vi "HEWH Gas Thermal Rate Tester.vi"() -> ()   [LabVIEW 2019]
uses:
  Type Definitions/HEWH Output Information.ctl
  Type Definitions/HEWH Draw Pattern Setup.ctl
  Type Definitions/PRAT Test.ctl
  Utility/Save File/File Setup (Public)/Type Definition/Save File HEWH Heating Control Mode.ctl
  Support VIs/Draw Water Specific/Type Definitions/Terminate Draw Conditions.ctl
  Type Definitions/HEWH Start Conditions.ctl
  Support VIs/Draw Water Specific/Type Definitions/Check Special Condtions.ctl
  Support VIs/Draw Water Specific/Type Definitions/HEWH Special Condition Check.ctl
  Type Definitions/HEWH Draw Flag ENUM.ctl
  Type Definitions/HEWH Specific DAQ.ctl
  Type Definitions/HEWH Power Data.ctl
  Type Definitions/HEWH Power Elements.ctl
  Utility/Type Definitions/UTILITY Power Analyzer.ctl
  Type Definitions/HEWH Calc and Calibration.ctl
  Utility/Save File/File Setup (Public)/Type Definition/Save File DOE LabView Program.ctl
  Custom Instrument Control/MW100/Type Definitions/Station ID Selector.ctl
  Range/Type Definitions/RANGE ANSI Rate.ctl
  Drivers/Alicat Gas Meter Driver/Sub-VIs/Data Cluster.ctl
  <vilib>/Utility/file.llb/Read Delimited Spreadsheet (string).vi
  Utility/Save File/File Setup.lvlib
panel:
  out "Target Flow Rate (GPM)":dbl
  out "States":T1(array[ring])
  in  "FileInit Cluster Input in":T2={"Scan Rate Adjust"=0.0, "Draw Count"=0, "Test Patten Setup"={"Total Gallons Schedule"=[], "PRAT/RLT Sequence"=[], "Current Sequence Index"=0}, "HEWH Specific DAQ"={"HEWH Data"={"HEWH Standard"={"Voltage (Volts)"=0.0, "Current (Amps)"=0.0, "Power (Watts)"=0.0, "WattHours (Wh)"=0.0, "TC Tree (AVG)"=0.0, "Flow Rate (GPM)"=0.0, "Gallons (Gal)"=0.0, "RTD Out (Deg F)"=0.0, "RTD In (Deg F)"=0.0, "RTD Amb (Deg F)"=0.0, "TC Down"=0.0, "UE Event Lead"=0, "LE Event Lead"=0, "TC Tree Array"=[]}, "PRAT"={"Power (Watts) A"=0.0, "Power (Watts) B"=0.0, "Power (Watts) C"=0.0, "Power (Watts) D"=0.0, "TC1"=0.0, "TC2"=0.0, "TC3"=0.0, "TC4"=0.0, "WattHours (Wh) A"=0.0, "WattHours (Wh) B"=0.0, "WattHours (Wh) C"=0.0, "WattHours (Wh) D"=0.0, "Ambient"=0.0, "Extra Temp"=0.0}, "Additional Power Data"={"Vthd"=0.0, "Frequency (Hz)"=0.0, "Apparent Power (VA)"=0.0, "Power Factor"=0.0, "Current Crest Factor"=0.0, "Voltage Crest Factor"=0.0, "Integration Time (sec)"=0.0}}, "Flow Valve % Open"=0.0, "Power State"={"UE"=FALSE, "LE"=FALSE, "COMP"=FALSE, "FANS"=FALSE}, "Power Analyzer"=enum."", "Flow Valve uA Output"=0, "Gallons Start (Gal)"=0.0}, "Test Output Data"={"PreDraw Data Table"=[], "Data Table"=[], "MW100 TC Headers"=[]}, "Calc and Calibration"={"Mean SD Var Max Min Array"=[], "Draw Statistics (DBL)"=[], "Calibration Coefficients DBL"=[], "Start Gallons"=0.0, "Starting Temp Decline"=0.0, "K-Factor (Temperature)"=0.0, "All Draw Stats"=[], "RTD Terminate Value"=0.0, "K-Factor (Flow)"=0.0, "Intellifaucet Type"="", "Gas Thermal Stabilization Array"=[], "Gas Thermal Stabil Complete"=FALSE, "Gas Thermal Time"=0.0, "Therm Reset Cmpt 1"=FALSE, "Therm Reset Cmpt 2"=FALSE, "Last Flow Rate (Therm)"=0.0, "State"=enum."State 1", "Gas Thermal Time 2"=0.0}, "Current Draw Time"=0.0, "LV Program"=enum."No Name Found", "Station ID"=enum."", "Current Cond"=enum."N/A", "Test Complete"=FALSE, "ANSI Rate"={"Array 1"=[], "Array 3"=[], "Array 2"=[], "Start ANSI"=FALSE, "ANSI Start Time"=0.0, "Restart ANSI"=FALSE, "15 Min ANSI Avg (BTU/hr)"=0.0, "20 Min ANSI Avg (BTU/hr)"=0.0, "25 Min ANSI Avg (BTU/hr)"=0.0, "Absolute Pressure"=0.0, "Gas Temperature"=0.0, "Volumetric Flow Rate"=0.0, "Mass Flow Rate"=0.0, "Array 4"=[], "Array 5"=[], "Gas Rate"=0.0, "15 Min Pres Avg (PSIA)"=0.0, "20 Min Pres Avg (PSIA)"=0.0, "25 Min Pres Avg (PSIA)"=0.0, "15 Min Temp Avg (°F) "=0.0, "20 Min Temp Avg (°F)"=0.0, "25 Min Temp Avg (°F)"=0.0, "15 Min Uncorrected Avg (CFH)"=0.0, "20 Min Uncorrected Avg (CFH)"=0.0, "25 Min Uncorrected Avg (CFH)"=0.0, "15 Min Corrected Avg (SCFH)"=0.0, "20 Min Corrected Avg (SCFH)"=0.0, "25 Min Corrected Avg (SCFH)"=0.0, "15 Min Complete"=FALSE, "20 Min Complete"=FALSE, "25 Min Complete"=FALSE, "Heating Value (BTU/ft³)"=0.0}, "Gas Measurment Data"={"Absolute Pressure"=0.0, "Gauge/Diff. Pressure"=0.0, "Barometric Pressure"=0.0, "Temperature"=0.0, "Volumetric Flow"=0.0, "Mass Flow"=0.0, "Setpoint"=0.0, "Valve Drive"=0.0, "Totalizer"=0.0, "[hr]"=0.0, "[min]"=0.0, "[sec]"=0.0, "Totalizer Average Flow"=0.0, "Totalizer Peak Flow"=0.0, "Gas selected"=""}} {"Test Patten Setup"."PRAT/RLT Sequence"."Time" format="%<%H:%M:%S>t"; "Test Patten Setup"."Total Gallons Schedule" format="%.2f"}
  in  "file path (dialog if empty)":path
  out "all rows":string[][](array[string])
  # "Totalizer Timer"
  # "Draw Pattern Setup (24 Hour)"
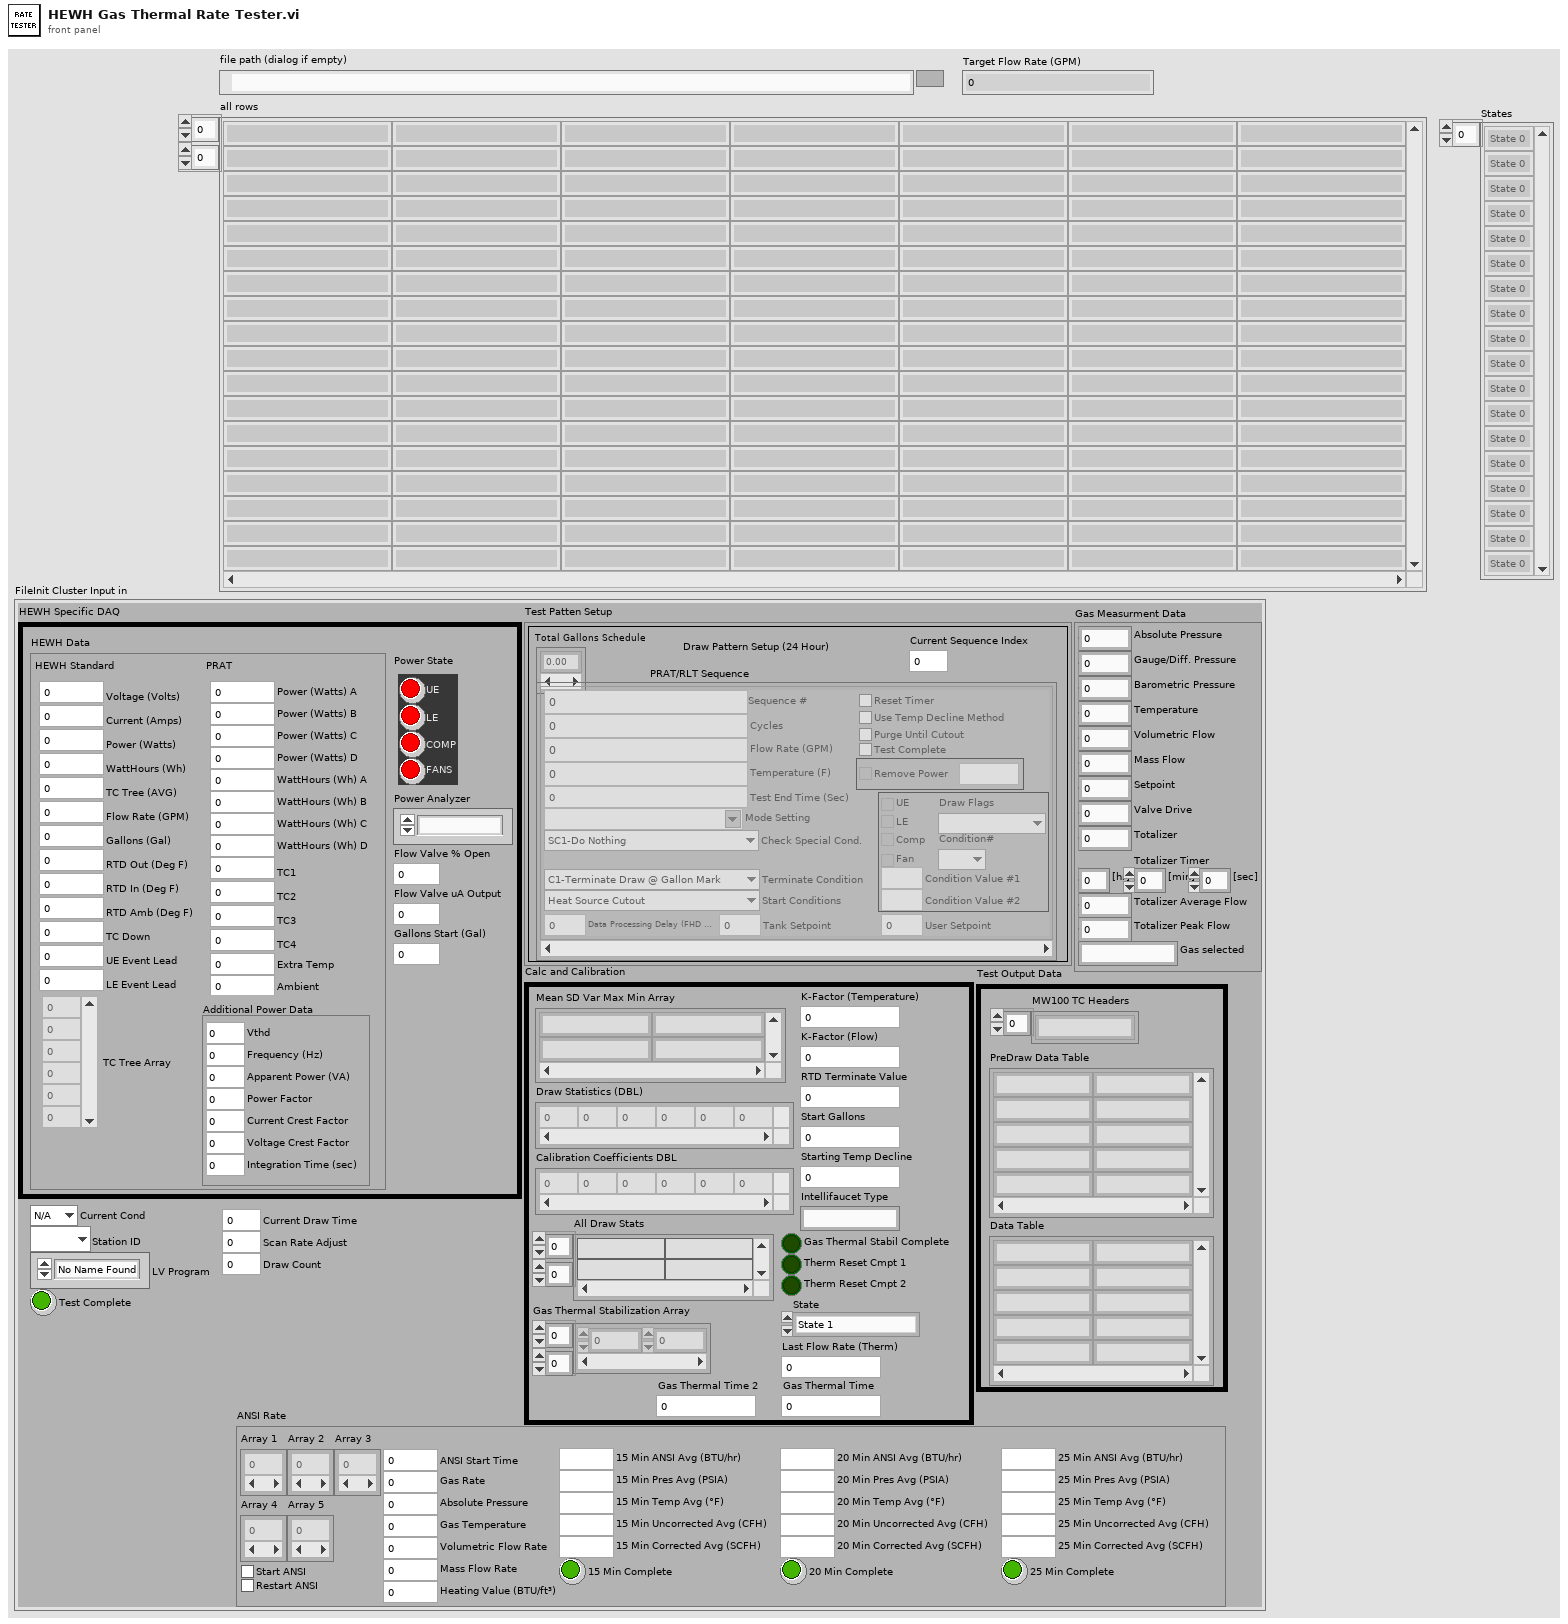
[diagram p1: front panel]
types:
  T1 = enum16{"State 0", "State 1", "State 2", "State 3", "State 4", "State 5"}[]
  T2 = typedef "HEWH Output Information.ctl" = cluster{"Scan Rate Adjust":dbl, "Draw Count":i32, "Test Patten Setup":T3, "HEWH Specific DAQ":T11, "Test Output Data":cluster{"PreDraw Data Table":string[][], "Data Table":string[][], "MW100 TC Headers":string[]}, "Calc and Calibration":T15, "Current Draw Time":dbl, "LV Program":T16, "Station ID":T17, "Current Cond":T9, "Test Complete":bool, "ANSI Rate":T18, "Gas Measurment Data":T19}
  T3 = typedef "HEWH Draw Pattern Setup.ctl" = cluster{"Total Gallons Schedule":dbl[], "PRAT/RLT Sequence":T4[], "Current Sequence Index":i32}
  T4 = typedef "PRAT Test.ctl" = cluster{"Sequence #":dbl, "Cycles":i32, "Mode Setting":T5, "Flow Rate (GPM)":dbl, "Temperature (F)":dbl, "Reset Timer":bool, "Use Temp Decline Method":bool, "Terminate Condition":T6, "Condition Value #1":dbl, "UE":bool, "LE":bool, "Comp":bool, "Fan":bool, "Test End Time (Sec)":dbl, "Purge Until Cutout":bool, "Start Conditions":T7, "Condition Value #2":dbl, "Remove Power":bool, "Time":dbl, "Check Special Cond.":T8, "Condition#":T9, "Draw Flags":T10, "Data Processing Delay (FHD 15sec, UEF 5 Sec)":dbl, "Test Complete":bool, "User Setpoint":dbl, "Tank Setpoint":dbl}
  T5 = typedef "File Setup.lvlib/Save File HEWH Heating Control Mode.ctl" = string
  T6 = typedef "Terminate Draw Conditions.ctl" = enum16{"C1-Terminate Draw @ Gallon Mark", "C2-Special Last Draw (HU Test)", "C3-RTD Out <=", "C4-Mean Tank Temp <=", "C5-Decrease RTD Out (Deg F)", "C6-Time (Seconds)", "C7-Until Any Heat Source", "C8-Specific Heat Source", "C9-Do Nothing", "C10-Inlet Outlet RTD Temp Delta"}
  T7 = typedef "HEWH Start Conditions.ctl" = enum16{"Heat Source Cutout", "At Time (Seconds)", "Every X (Seconds)", "T2 >= X° Below Setpoint", "Seconds From Complete", "Wait for LE & Comp Cutout", "Wait for Comp Cutout", "Wait for LE Cutout", "Wait for UE Cutout", "Start Immediately"}
  T8 = typedef "Check Special Condtions.ctl" = enum16{"SC1-Do Nothing", "SC2-Check Heat Source (On-C2/Off-C1)", "SC3-Check Skip Condition", "SC4-Check Heat Source ON/Fail", "SC5-Keep Draw Valves Open", "SC6-Skip Purge"}
  T9 = typedef "HEWH Special Condition Check.ctl" = enum16{"N/A", "C1", "C2", "Reset/Fail", "Skip Draw Sequence"}
  T10 = typedef "HEWH Draw Flag ENUM.ctl" = enum16{"N/A", "None(0)", "Sml(1)", "Med(2)", "SmlMed(3)", "Lrg(4)", "SmlLrg(5)", "MedLrg(6)", "SmlMedLrg(7)"}
  T11 = typedef "HEWH Specific DAQ.ctl" = cluster{"HEWH Data":T12, "Flow Valve % Open":dbl, "Power State":T13, "Power Analyzer":T14, "Flow Valve uA Output":i32, "Gallons Start (Gal)":dbl}
  T12 = typedef "HEWH Power Data.ctl" = cluster{"HEWH Standard":cluster{"Voltage (Volts)":dbl, "Current (Amps)":dbl, "Power (Watts)":dbl, "WattHours (Wh)":dbl, "TC Tree (AVG)":dbl, "Flow Rate (GPM)":dbl, "Gallons (Gal)":dbl, "RTD Out (Deg F)":dbl, "RTD In (Deg F)":dbl, "RTD Amb (Deg F)":dbl, "TC Down":dbl, "UE Event Lead":i32, "LE Event Lead":i32, "TC Tree Array":dbl[]}, "PRAT":cluster{"Power (Watts) A":dbl, "Power (Watts) B":dbl, "Power (Watts) C":dbl, "Power (Watts) D":dbl, "TC1":dbl, "TC2":dbl, "TC3":dbl, "TC4":dbl, "WattHours (Wh) A":dbl, "WattHours (Wh) B":dbl, "WattHours (Wh) C":dbl, "WattHours (Wh) D":dbl, "Ambient":dbl, "Extra Temp":dbl}, "Additional Power Data":cluster{"Vthd":dbl, "Frequency (Hz)":dbl, "Apparent Power (VA)":dbl, "Power Factor":dbl, "Current Crest Factor":dbl, "Voltage Crest Factor":dbl, "Integration Time (sec)":dbl}}
  T13 = typedef "HEWH Power Elements.ctl" = cluster{"UE":bool, "LE":bool, "COMP":bool, "FANS":bool}
  T14 = typedef "UTILITY Power Analyzer.ctl" = enum16{"", "APLUS", "WT210", "WT500", "WT300", "OSI", "Debug", "WT230", "WT300_1", "WT300_2"}
  T15 = typedef "HEWH Calc and Calibration.ctl" = cluster{"Mean SD Var Max Min Array":string[][], "Draw Statistics (DBL)":dbl[][], "Calibration Coefficients DBL":dbl[][], "Start Gallons":dbl, "Starting Temp Decline":dbl, "K-Factor (Temperature)":dbl, "All Draw Stats":string[][], "RTD Terminate Value":dbl, "K-Factor (Flow)":dbl, "Intellifaucet Type":string, "Gas Thermal Stabilization Array":dbl[][], "Gas Thermal Stabil Complete":bool, "Gas Thermal Time":dbl, "Therm Reset Cmpt 1":bool, "Therm Reset Cmpt 2":bool, "Last Flow Rate (Therm)":dbl, "State":enum16{"State 0", "State 1", "State 2", "State 3", "State 4", "State 5"}, "Gas Thermal Time 2":dbl}
  T16 = typedef "File Setup.lvlib/Save File DOE LabView Program.ctl" = enum16{"No Name Found", "DOE Stand", "Dishwasher Kitchen", "Portable Stand", "HEWH", "Dryer", "Dryer WILT", "HCC", "PRAT", "HEWH RLT", "Refrigeration", "Gas Water Heater"}
  T17 = typedef "Station ID Selector.ctl" = enum16{"", "A", "B", "C", "D", "Global"}
  T18 = typedef "RANGE ANSI Rate.ctl" = cluster{"Array 1":dbl[], "Array 3":dbl[], "Array 2":dbl[], "Start ANSI":bool, "ANSI Start Time":dbl, "Restart ANSI":bool, "15 Min ANSI Avg (BTU/hr)":dbl, "20 Min ANSI Avg (BTU/hr)":dbl, "25 Min ANSI Avg (BTU/hr)":dbl, "Absolute Pressure":dbl, "Gas Temperature":dbl, "Volumetric Flow Rate":dbl, "Mass Flow Rate":dbl, "Array 4":dbl[], "Array 5":dbl[], "Gas Rate":dbl, "15 Min Pres Avg (PSIA)":dbl, "20 Min Pres Avg (PSIA)":dbl, "25 Min Pres Avg (PSIA)":dbl, "15 Min Temp Avg (°F) ":dbl, "20 Min Temp Avg (°F)":dbl, "25 Min Temp Avg (°F)":dbl, "15 Min Uncorrected Avg (CFH)":dbl, "20 Min Uncorrected Avg (CFH)":dbl, "25 Min Uncorrected Avg (CFH)":dbl, "15 Min Corrected Avg (SCFH)":dbl, "20 Min Corrected Avg (SCFH)":dbl, "25 Min Corrected Avg (SCFH)":dbl, "15 Min Complete":bool, "20 Min Complete":bool, "25 Min Complete":bool, "Heating Value (BTU/ft³)":dbl}
  T19 = typedef "Data Cluster.ctl" = cluster{"Absolute Pressure":dbl, "Gauge/Diff. Pressure":dbl, "Barometric Pressure":dbl, "Temperature":dbl, "Volumetric Flow":dbl, "Mass Flow":dbl, "Setpoint":dbl, "Valve Drive":dbl, "Totalizer":dbl, "[hr]":dbl, "[min]":dbl, "[sec]":dbl, "Totalizer Average Flow":dbl, "Totalizer Peak Flow":dbl, "Gas selected":string}
  T20 = enum16{"State 0", "State 1", "State 2", "State 3", "State 4", "State 5"}
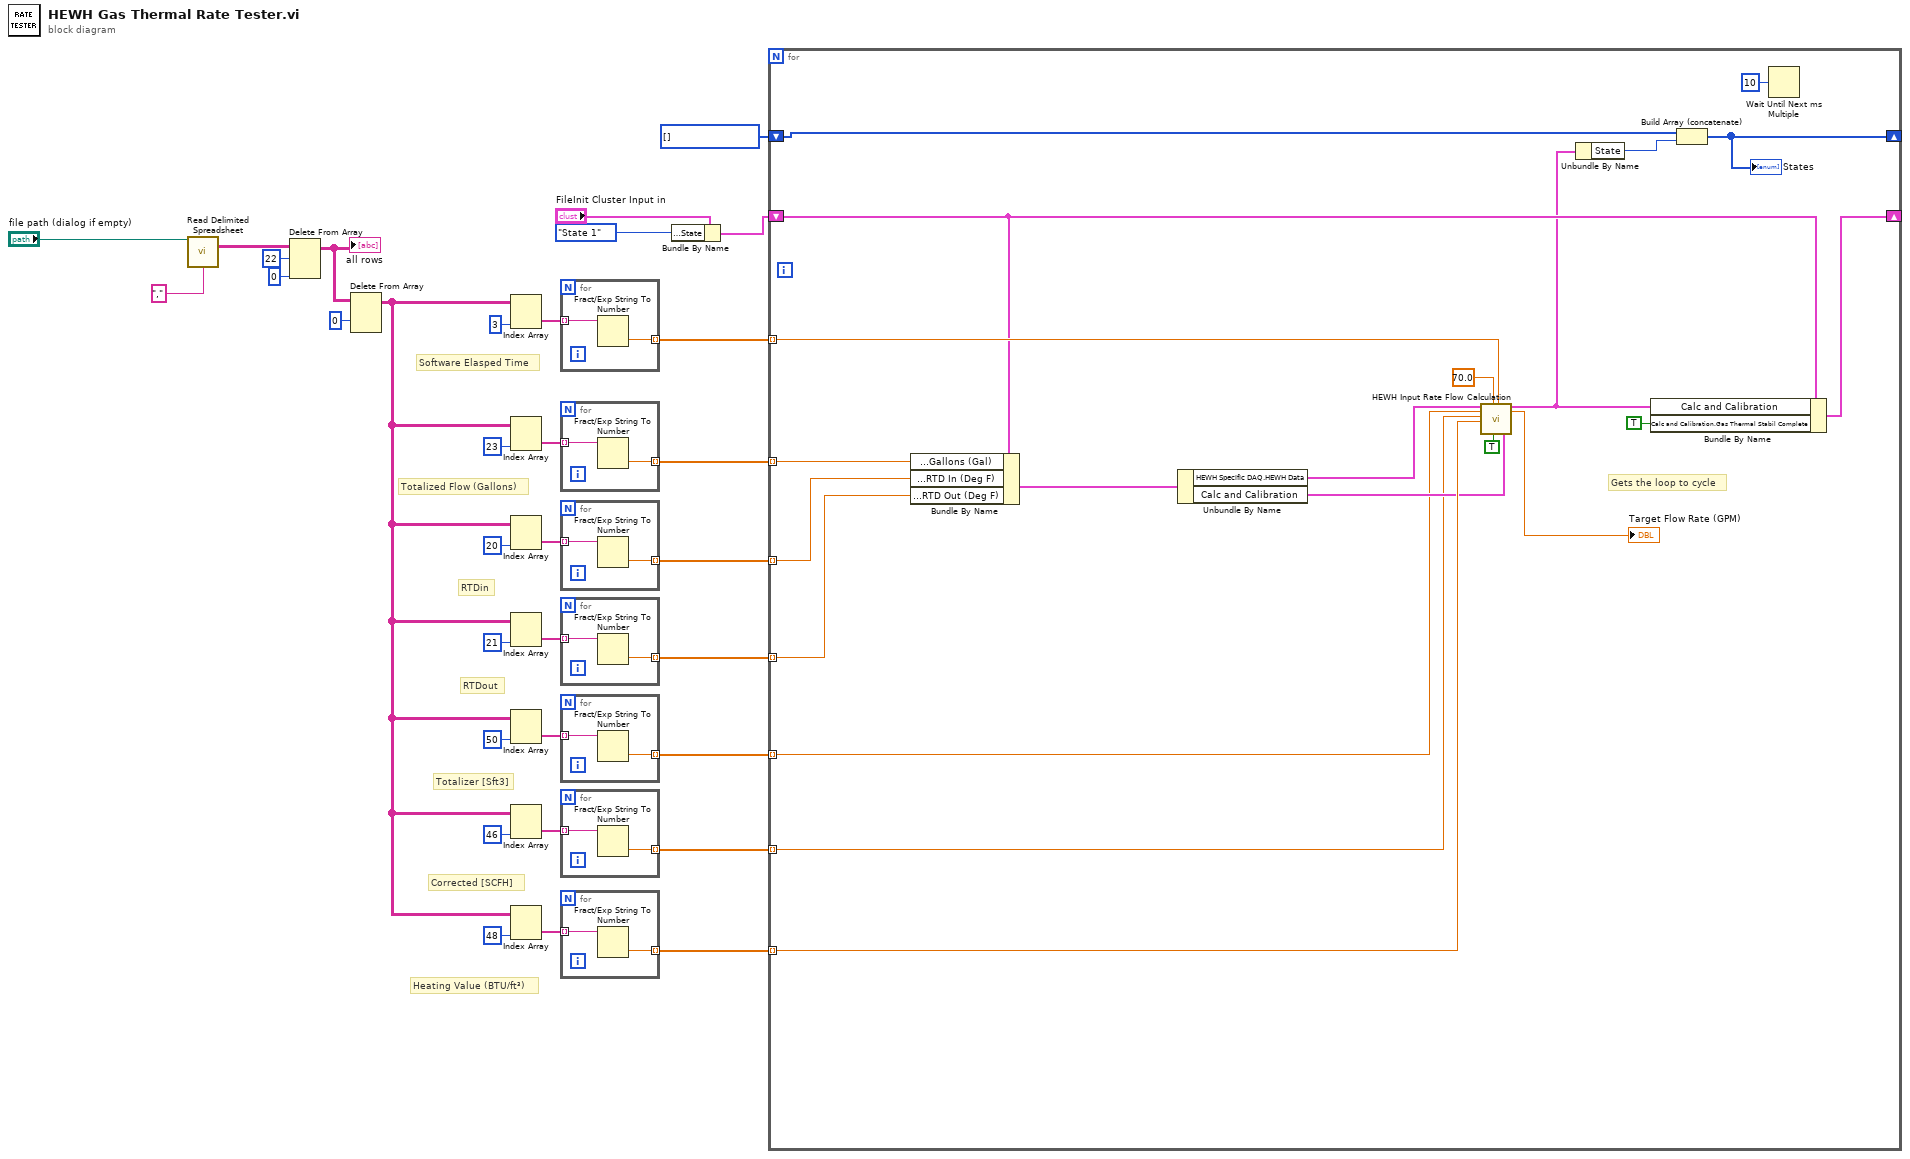
[diagram p0: block diagram]
diagram:
  w1 = T1 [] items=["State 0", "State 1", "State 2", "State 3", "State 4", "State 5"]
  # "Corrected [SCFH]"
  # "Totalizer [Sft3]"
  # "Totalized Flow (Gallons)"
  # "Heating Value (BTU/ft³)"
  # "RTDout"
  # "RTDin"
  # "Software Elasped Time"
  n1 = call-poly <vilib>:"Read Delimited Spreadsheet.vi"("file path (dialog if empty)"="file path (dialog if empty)", "delimiter (\\t)"="," ("delimiter (\\t)")) -> ("all rows"=w23:string[][])  [unwired: 8 in, 5 out]
  n2 = Delete From Array(array=w23, length=22, index (row)=0) -> (array with subset deleted=w26:string[][])  [unwired: 1 in, 1 out]
  "all rows" <- w26
  n3 = Delete From Array(array=w26, index (row)=0) -> (array with subset deleted=w6:string[][])  [unwired: 2 in, 1 out]
  n4 = Index Array(array=w6, index (col)=3 ("disabled index (col)")) -> (element=w28:string[])  [unwired: 1 in]
  n5 = Index Array(array=w6, index (col)=23 ("disabled index (col)")) -> (element=w16:string[])  [unwired: 1 in]
  n6 = Index Array(array=w6, index (col)=20 ("disabled index (col)")) -> (element=w32:string[])  [unwired: 1 in]
  n7 = Index Array(array=w6, index (col)=21 ("disabled index (col)")) -> (element=w33:string[])  [unwired: 1 in]
  n8 = Index Array(array=w6, index (col)=50 ("disabled index (col)")) -> (element=w11:string[])  [unwired: 1 in]
  n9 = Index Array(array=w6, index (col)=46 ("disabled index (col)")) -> (element=w7:string[])  [unwired: 1 in]
  n10 = Index Array(array=w6, index (col)=48 ("disabled index (col)")) -> (element=w19:string[])  [unwired: 1 in]
  n11 = for {
    tunnel: w28 -> [w35] mode=indexing
    tunnel: [w34] -> w17 mode=indexing
    n12 = Fract/Exp String To Number(string=w35) -> (number=w34:dbl)  [unwired: 3 in, 1 out]
  }
  n13 = for {
    tunnel: w16 -> [w37] mode=indexing
    tunnel: [w36] -> w14 mode=indexing
    n14 = Fract/Exp String To Number(string=w37) -> (number=w36:dbl)  [unwired: 3 in, 1 out]
  }
  n15 = for {
    tunnel: w32 -> [w39] mode=indexing
    tunnel: [w38] -> w13 mode=indexing
    n16 = Fract/Exp String To Number(string=w39) -> (number=w38:dbl)  [unwired: 3 in, 1 out]
  }
  n17 = for {
    tunnel: w33 -> [w41] mode=indexing
    tunnel: [w40] -> w12 mode=indexing
    n18 = Fract/Exp String To Number(string=w41) -> (number=w40:dbl)  [unwired: 3 in, 1 out]
  }
  n19 = for {
    tunnel: w11 -> [w43] mode=indexing
    tunnel: [w42] -> w9 mode=indexing
    n20 = Fract/Exp String To Number(string=w43) -> (number=w42:dbl)  [unwired: 3 in, 1 out]
  }
  n21 = for {
    tunnel: w7 -> [w45] mode=indexing
    tunnel: [w44] -> w5 mode=indexing
    n22 = Fract/Exp String To Number(string=w45) -> (number=w44:dbl)  [unwired: 3 in, 1 out]
  }
  n23 = for {
    tunnel: w19 -> [w47] mode=indexing
    tunnel: [w46] -> w18 mode=indexing
    n24 = Fract/Exp String To Number(string=w47) -> (number=w46:dbl)  [unwired: 3 in, 1 out]
  }
  n25 = Bundle By Name(cluster="FileInit Cluster Input in", "Calc and Calibration.State"=T20."State 1") -> (w3:T2)
  n26 = for {
    tunnel: w18 -> [w68] mode=indexing
    tunnel: w17 -> [w65] mode=indexing
    tunnel: w14 -> [w64] mode=indexing
    tunnel: w13 -> [w63] mode=indexing
    tunnel: w12 -> [w62] mode=indexing
    tunnel: w9 -> [w58] mode=indexing
    tunnel: w5 -> [w51] mode=indexing
    shift-right: [w56] -> _
    shift-left: w3 -> [w57]
    shift-right: [w52] -> _
    shift-left: w1 -> [w53]
    # "Gets the loop to cycle"
    n27 = Bundle By Name(cluster=w57, "HEWH Specific DAQ.HEWH Data.HEWH Standard.Gallons (Gal)"=w64, "HEWH Specific DAQ.HEWH Data.HEWH Standard.RTD In (Deg F)"=w63, "HEWH Specific DAQ.HEWH Data.HEWH Standard.RTD Out (Deg F)"=w62) -> (w61:T2)
    n28 = Unbundle By Name(w61) -> ("HEWH Specific DAQ.HEWH Data"=w60:T12, "Calc and Calibration"=w59:T15)
    n29 = call "HEWH Input Rate Flow Calculation.vi"("HEWH Data"=w60, "Totalizer (Debug)"=w58, "Mass Flow (Debug)"=w51, "Heating Value (BTU/ft³)"=w68, "Delta T Target"=70.0, "Debug"=TRUE, "Elapsed Time (sec)"=w65, "Calc and Calibration"=w59) -> ("Calc and Calibration Output"=w55:T15, "Target Flow Rate (GPM)"=→"Target Flow Rate (GPM)":dbl)  [unwired: 9 in, 1 out]
    n30 = Unbundle By Name(w55) -> ("State"=w54:T20)
    n31 = Bundle By Name(cluster=w57, "Calc and Calibration"=w55, "Calc and Calibration.Gas Thermal Stabil Complete"=TRUE) -> (w56:T2)
    n32 = Build Array (concatenate)(w53, w54) -> (w52:T1)
    "States" <- w52
    n33 = Wait Until Next ms Multiple(millisecond multiple=u32 10) -> ()  [unwired: 1 out]
  }
